vi "Parse POTCAR.vi"(8 "error in (no error)":errorcluster, 11 "POTCAR File":path=path "C:/Users/Chris B/Documents/Ab Initio/Vasp Calculations/Batch4_20130519/1_Again") -> (0 "error out":errorcluster, 3 "POTCARs":string[](array[string]))   [LabVIEW 2010]
uses:
  <vilib>/regexp/Match Regular Expression.xnode
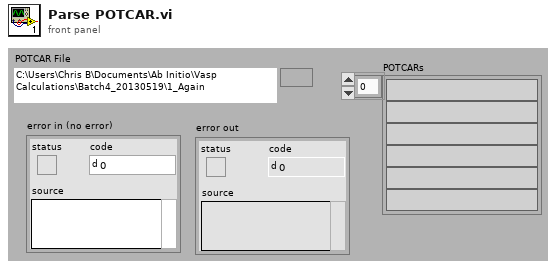
[diagram p1: front panel]
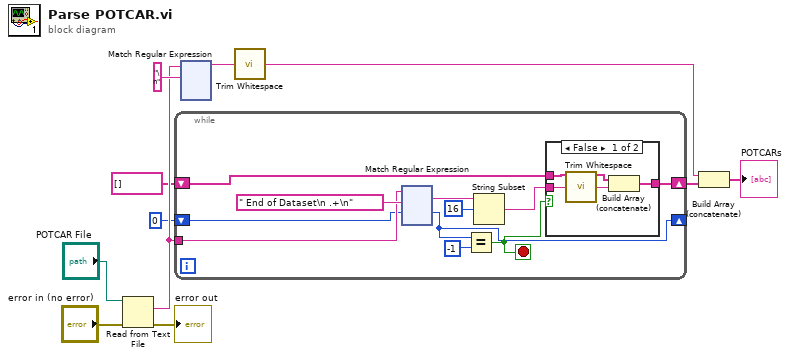
[diagram p0: block diagram]
diagram:
  n1 = Read from Text File(file (use dialog)="POTCAR File", error in="error in (no error)") -> (text=w6:string, error out=→"error out":errorcluster)  [unwired: 2 in, 2 out]
  n2 = while {
    shift-right: [w16] -> _
    shift-left: 0 ("offset past match") -> [w17]
    tunnel: w6 -> [w18]
    shift-right: [w12] -> w3
    shift-left: string[] [] -> [w13]
    stop <- w15 stop-if-true
    n3 = xnode "Match Regular Expression"("input string"=w18, "regular expression"=" End of Dataset\n .+\n", "offset (0)"=w17) -> ("whole match"=w21:string, "offset past match"=w16:i32)  [unwired: 3 in, 3 out]
    n4 = Equal?(x=w16, y=-1) -> (x = y?=w15:bool)
    n5 = String Subset(string=w21, offset (0)=16) -> (substring=w14:string)  [unwired: 1 in]
    n6 = case shown="False" w15 {
      tunnel: w14 -> [w24 _]
      tunnel: [w26 w27] -> w12
      tunnel: w13 -> [w25 w27]
      frame False {
        n7 = call <vilib>:"Trim Whitespace.vi"("string"=w24) -> ("trimmed string"=w23:string)  [unwired: 1 in]
        n8 = Build Array (concatenate)(w25, w23) -> (w26:string[])
      }
      frame True {
      }
    }
  }
  n9 = xnode "Match Regular Expression"("input string"=w6, "regular expression"="\n") -> ("before match"=w8:string)  [unwired: 4 in, 4 out]
  n10 = call <vilib>:"Trim Whitespace.vi"("string"=w8) -> ("trimmed string"=w7:string)  [unwired: 1 in]
  n11 = Build Array (concatenate)(w7, w3) -> (→"POTCARs":string[])
